vi "ShooterTest.vi"() -> ()   [LabVIEW 2013]
uses:
  <vilib>/Rock Robotics/SystemInterfaces/Typedef/FPGA_TypedefSolenoidModule.ctl
  <vilib>/Rock Robotics/WPI/Solenoid/WPI_SolenoidChannel.ctl
  Robot_Framework_2014/SingleSolenoidAction.ctl
  <vilib>/Rock Robotics/WPI/Joystick/WPI_JoystickDeviceEnum.ctl
  <vilib>/Rock Robotics/WPI/Solenoid/WPI_SolenoidOpenSingle.vi
panel:
  in  "Kicker Module":T1
  in  "Kicker Channel":T2
  in  "Firing Channel":T2
  in  "Firing Module":T1
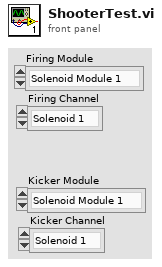
[diagram p1: front panel]
types:
  T1 = typedef "FPGA_TypedefSolenoidModule.ctl" = enum16{"Solenoid Module 1", "Solenoid Module 2"}
  T2 = typedef "WPI_SolenoidChannel.ctl" = enum8{"Solenoid 1", "Solenoid 2", "Solenoid 3", "Solenoid 4", "Solenoid 5", "Solenoid 6", "Solenoid 7", "Solenoid 8", "Invalid"}
  T3 = typedef "WPI_JoystickDeviceEnum.ctl" = enum16{"USB 1", "USB 2", "USB 3", "USB 4", "Kinect 1", "Kinect 2"}
  T4 = typedef "SingleSolenoidAction.ctl" = enum16{"Init", "SetState", "Disable"}
  T5 = typedef "WPI_JoystickDevRef.ctl" = cluster{"Device":T3}
  T6 = typedef "WPI_SolenoidDevRef.ctl" = cluster{"DevStatus":errorcluster, "Solenoid Module":T1, "Forward Solenoid Channel":T2, "Reverse Solenoid Channel":T2}
  T7 = typedef "WPI_JoystickButtonState.ctl" = cluster{"Button 1":bool, "Button 2":bool, "Button 3":bool, "Button 4":bool, "Button 5":bool, "Button 6":bool, "Button 7":bool, "Button 8":bool, "Button 9":bool, "Button 10":bool, "Button 11":bool, "Button 12":bool}
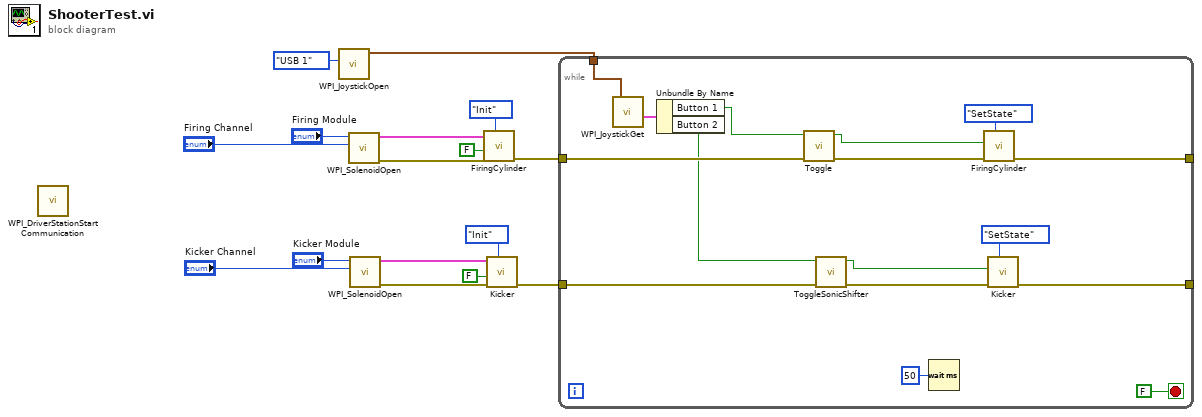
[diagram p0: block diagram]
diagram:
  n1 = call <vilib>:"WPI_DriverStationStart Communication.vi"() -> ()  [unwired: 12 in]
  n2 = call <vilib>:"WPI_JoystickOpen.vi"("JoystickDevice"=WPI_JoystickDeviceEnum."USB 1") -> ("JoystickDevRef"=w2:T5)  [unwired: 10 in]
  n3 = call-poly <vilib>:"WPI_SolenoidOpen.vi"("Solenoid Channel"="Firing Channel", "Solenoid Module (Module 1)"="Firing Module") -> ("error out"=w4:errorcluster, "SolenoidDevRef"=w5:T6)  [unwired: 8 in]
  n4 = call-poly <vilib>:"WPI_SolenoidOpen.vi"("Solenoid Channel"="Kicker Channel", "Solenoid Module (Module 1)"="Kicker Module") -> ("error out"=w3:errorcluster, "SolenoidDevRef"=w6:T6)  [unwired: 8 in]
  n5 = call "FiringCylinder.vi"("Action"=SingleSolenoidAction."Init", "error in (no error)"=w4, "Default Position"=FALSE, "SolenoidDevRef"=w5) -> ("error out"=w14:errorcluster)  [unwired: 7 in]
  n6 = call "Kicker.vi"("Action"=SingleSolenoidAction."Init", "error in (no error)"=w3, "Default Position"=FALSE, "SolenoidDevRef"=w6) -> ("error out"=w13:errorcluster)  [unwired: 7 in]
  n7 = while {
    tunnel: [w28] -> _
    tunnel: [w27] -> _
    tunnel: w14 -> [w26]
    tunnel: w13 -> [w25]
    tunnel: w2 -> [w24]
    stop <- FALSE stop-if-true
    n8 = call <vilib>:"WPI_JoystickGet.vi"("JoystickDevRef"=w24) -> ("Buttons"=w22:T7)  [unwired: 4 in, 2 out]
    n9 = Unbundle By Name(w22) -> ("Button 1"=w21:bool, "Button 2"=w19:bool)
    n10 = call "Toggle.vi"("error in"=w26, "RawInput"=w21) -> ("error out"=w23:errorcluster, "ToggleState"=w17:bool)  [unwired: 8 in]
    n11 = call "ToggleSonicShifter.vi"("error in"=w25, "cSonicShifter"=w19) -> ("error out"=w20:errorcluster, "Actuate?"=w18:bool)  [unwired: 8 in]
    n12 = Wait (ms)(milliseconds to wait=u32 50) -> ()  [unwired: 1 out]
    n13 = call "FiringCylinder.vi"("Action"=SingleSolenoidAction."SetState", "error in (no error)"=w23, "Actuate?"=w17) -> ("error out"=w27:errorcluster)  [unwired: 8 in]
    n14 = call "Kicker.vi"("Action"=SingleSolenoidAction."SetState", "error in (no error)"=w20, "Actuate?"=w18) -> ("error out"=w28:errorcluster)  [unwired: 8 in]
  }
